vi "Constructor.vi"(8 "error in (no error)":errorcluster, 11 "Valve Controller in":refnum<class "Valve Controller.lvclass">) -> (0 "error out":errorcluster, 2 "Init":bool, 3 "Valve Controller out":refnum<class "Valve Controller.lvclass">)   [LabVIEW 2011, in "Valve Controller.lvclass"]
uses:
  Valve Controller.lvclass
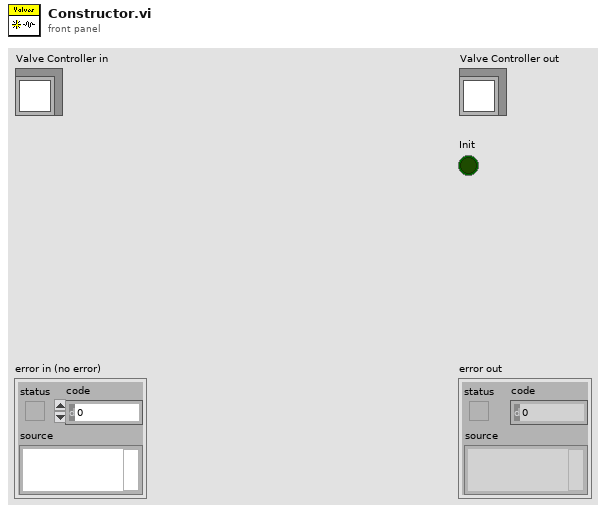
[diagram p1: front panel]
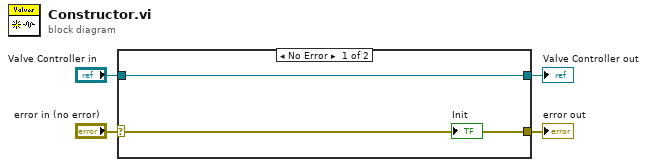
[diagram p0: block diagram]
diagram:
  n1 = case shown="No Error" "error in (no error)" {
    selector: "error in (no error)" -> [w5 w8]
    tunnel: [w5 w8] -> w3
    tunnel: [w6 w7] -> w1
    tunnel: "Valve Controller in" -> [w6 w7]
    frame No Error {
    }
    frame Error {
    }
  }
  "error out" <- w3
  "Valve Controller out" <- w1
